vi "geis.vi"(0 "IP adress":string="192.109.209.229", 1 "stop":bool, 2 "Channel":u8(ring) items=["1", "2", "3", "4", "5", "6", "7", "8", "9", "10", "11", "12", "13", "14", "15", "16"], 3 "SGEIS Parameters":T2={"Step_number"=0, "Initial_Current_step"=0.0, "vs_initial "=TRUE, "Final_Current_step"=0.001, "vs_final"=TRUE, "Duration_step"=1.0, "Record_every_dE"=0.1, "Record_every_dT"=0.1, "Initial_frequency"=100000.0, "sweep"=FALSE, "Final_frequency"=1.0, "Frequency_number"=51, "Amplitude_Current"=0.001, "Wait_for_steady"=2.0, "Average_N_times"=1, "Correction"=TRUE, "I_Range"=7, "Bandwidth"=5, "Initial_Current_step 2"=0.01, "vs_initial 2"=FALSE, "em"=1, "ce"=0} {"ce" items=["Standard", "CE to ground"]; "Initial_Current_step" min=-10 max=10 format="%.5f"; "Step_number" min=0 step=1; "Initial_Current_step 2" min=-10 max=10 format="%.5f"; "I_Range" items=["1pA", "1nA", "10nA", "100nA", "1µA", "10µA", "100µA", "1mA", "10mA", "100mA", "1A", "Booster"]; "Bandwidth" items=["1"=1, "2"=2, "3"=3, "4"=4, "5"=5, "6"=6, "7"=7, "8"=8, "9"=9]; "Wait_for_steady" min=0 format="%.2f"; "Record_every_dT" min=0 format="%.2e"; "Record_every_dE" min=0 format="%.2e"; "Duration_step" min=0 format="%.5f"; "Final_Current_step" min=-10 max=10 format="%.5f"; "Average_N_times" min=1 max=1000 step=1; "Amplitude_Current" min=0 max=100 format="%.2e"; "Final_frequency" min=1e-05 max=1000000 format="%.2e"; "Frequency_number" min=1 max=10000; "Initial_frequency" min=1e-05 max=1000000 format="%.2e"}, 4 "Exit":bool, 5 "Start":bool, 8 "Draw":T1(ring)) -> (6 "Number of points":i32=52, 7 "XY Graph":cluster{"Data p1":sgl[], "Data p1":dbl[]}[](graph))   [LabVIEW 2012]
doc: "The Staircase Galvano Electrochemical Impedance Spectroscopy (SGEIS) technique is close to the SPEIS technique, except that the current is controlled instead of the potential.\n\nIn general, in this VI, the first thing to do is to start by establishing the connection with the instrument defined by its IP adress, then load the firmware in the channel selected, get the information on the plugged channels, load protocol on a channel, start/stop the protocol, retreive data and draw the graph.\nThis technique is applied just for channels with impedance capabilities (Zboard)."
uses:
  base_xml.llb/Type Descriptor Enumeration__ogtk.ctl
panel:
  out "Data P0":sgl[][](array[numeric])=[[4.8e-05, 1.2033013, 0.0012545494], [7.2e-05, 4.099232, 0.0030298461], [9.6e-05, 5.4905596, 0.0034574724], [0.00040800002, 5.594096, 0.0031739129], [0.00086400006, 5.697314, 0.00286901], [0.0014160001, 5.800989, 0.0025610582], [0.002112, 5.903515, 0.002253106], [0.0030480002, 6.0050545, 0.0019497279], [0.0045120004, 6.105221, 0.0016379646], [0.008280001, 6.2053866, 0.0013155299], [0.100008, 6.222552, 0.0012118629], [0.200016, 6.223086, 0.0012103383], [0.300024, 6.223086, 0.0012126251], [0.400032, 6.2233143, 0.0012133875], [0.50004, 6.2231617, 0.0012141496], [0.600048, 6.2229333, 0.0012133875], [0.700056, 6.2229333, 0.0012103383], [0.800064, 6.2227044, 0.0012095761], [0.90007204, 6.2233143, 0.0012149118]]
  out "Data P1":sgl[][](array[numeric])=[[99999.99, 0.015896028, 2.4134535e-05, -0.31541085, 6.2027836, 0.0012093844, 0.0, 0.028001478, 2.4202996e-05, -0.21167731, -6.8013325, -0.001209385, 0.0, 1.296, 8.0], [79789.055, 0.020694803, 3.145496e-05, -0.31517792, 6.1967587, 0.0012085777, 0.0, 0.036134787, 3.1510877e-05, -0.20527963, -6.7949142, -0.0012085784, 0.0, 1.584, 8.0], [63671.867, 0.027115118, 3.95239e-05, -0.36039186, 6.1889963, 0.0012069115, 0.0, 0.04638151, 3.95688e-05, -0.23149349, -6.7864842, -0.0012069122, 0.0, 1.872, 8.0], [50804.684, 0.035882276, 4.949095e-05, -0.40444195, 6.178996, 0.0012048192, 0.0, 0.05973892, 4.952679e-05, -0.25926352, -6.77554, -0.0012048199, 0.0, 2.16, 8.0], [40539.06, 0.048188828, 6.136454e-05, -0.4440093, 6.1657524, 0.0012020994, 0.0, 0.077702746, 6.139315e-05, -0.28762102, -6.7610307, -0.0012021001, 0.0, 2.448, 8.0], [32343.752, 0.06770085, 7.88223e-05, -0.47251844, 6.1465006, 0.0011982684, 0.0, 0.10554845, 7.884587e-05, -0.31181583, -6.739913, -0.0011982691, 0.0, 2.736, 8.0], [25812.496, 0.12644306, 0.0001329111, -0.48514298, 6.0997047, 0.0011887155, 0.0, 0.19051811, 0.00013293685, -0.32698154, -6.6886125, -0.0011887162, 0.0, 3.024, 8.0], [20593.748, 0.23297587, 0.00022114319, -0.47706103, 6.015843, 0.0011718888, 0.0, 0.34030145, 0.00022117054, -0.3275948, -6.596549, -0.0011718895, 0.0, 3.312, 8.0], [16429.69, 0.37617812, 0.00032387703, -0.45101714, 5.8985395, 0.0011485365, 0.0, 0.5348972, 0.00032390282, -0.31515712, -6.4677424, -0.0011485372, 0.0, 3.6000001, 8.0], [13109.373, 0.55603534, 0.00044012873, -0.4103434, 5.7451816, 0.0011180385, 0.0, 0.7737537, 0.00044015126, -0.2906543, -6.299325, -0.0011180392, 0.0, 3.888, 8.0], [10460.936, 0.7749276, 0.00057313335, -0.36184657, 5.5526934, 0.001079828, 0.0, 1.0605142, 0.0005731519, -0.25886726, -6.0878835, -0.0010798287, 1.0, 4.176, 8.0], [8351.5625, 1.0352163, 0.00072714745, -0.31150156, 5.3164287, 0.0010371187, 1.0, 1.3994575, 0.0007271621, -0.22451091, -5.8299828, -0.0010371194, 1.0, 4.609, 8.0], [6660.1553, 1.3410046, 0.000907536, -0.26282227, 5.0436444, 0.0009789959, 1.0, 1.7970788, 0.00090754736, -0.19028175, -5.5293727, -0.0009789965, 2.0, 4.947, 8.0], [5313.953, 1.5113798, 0.0009967732, -0.21961367, 4.8940244, 0.0009556693, 1.0, 2.0129824, 0.000996781, -0.15885389, -5.3671427, -0.00095566985, 2.0, 5.57, 8.0], [4241.786, 1.5454612, 0.0010015898, -0.18297291, 4.878454, 0.0009537674, 1.0, 2.0500069, 0.0010015944, -0.13264023, -5.3505425, -0.0009537679, 2.0, 6.213, 8.0], [3385.4163, 1.5790181, 0.0010115571, -0.153041, 4.8648095, 0.00095176516, 1.0, 2.0889149, 0.0010115607, -0.111195564, -5.3358197, -0.0009517657, 2.0, 6.857, 8.0], [2699.3184, 1.5802759, 0.0010046018, -0.1293776, 4.883166, 0.0009544167, 1.0, 2.0867875, 0.0010046042, -0.09421384, -5.3556128, -0.0009544172, 2.0, 7.501, 8.0], [2153.4448, 1.5856456, 0.001002952, -0.11168504, 4.8972144, 0.0009564839, 1.0, 2.0912726, 0.0010029528, -0.08150327, -5.370766, -0.0009564844, 2.0, 8.1449995, 8.0], [1717.748, 1.5895984, 0.0010019304, -0.09921706, 4.9112163, 0.0009589054, 1.0, 2.0948448, 0.0010019315, -0.072561264, -5.38597, -0.0009589059, 2.0, 8.792, 8.0], [1372.1951, 1.5920151, 0.0010009218, -0.09178877, 4.924607, 0.0009613617, 1.0, 2.0966747, 0.0010009219, -0.06731814, -5.400561, -0.0009613622, 2.0, 9.439, 8.0], [1096.7545, 1.6009942, 0.0010047532, -0.08871567, 4.9333324, 0.000961253, 1.0, 2.1073825, 0.001004754, -0.06525302, -5.4094787, -0.00096125354, 2.0, 9.871, 8.0], [871.93097, 1.5816059, 0.0009906995, -0.09027839, 4.959241, 0.000966918, 1.0, 2.0806665, 0.0009906992, -0.06663093, -5.4381466, -0.00096691854, 2.0, 10.307, 8.0], [696.1138, 1.5729876, 0.0009832102, -0.09623489, 4.9737277, 0.0009698118, 1.0, 2.0679011, 0.0009832109, -0.07122159, -5.454079, -0.0009698124, 2.0, 10.741, 8.0], [555.8894, 1.6019666, 0.0009985057, -0.106960624, 4.9539285, 0.00096688373, 1.0, 2.1039863, 0.0009985064, -0.07941079, -5.4326506, -0.0009668843, 2.0, 11.394, 8.0], [443.43906, 1.6082691, 0.0009985616, -0.122988224, 4.9526095, 0.0009666943, 1.0, 2.1093283, 0.000998562, -0.091551304, -5.4311996, -0.00096669485, 2.0, 12.053, 8.0], [353.75473, 1.6163155, 0.0009975499, -0.14474046, 4.9489985, 0.00096599624, 1.0, 2.1154938, 0.0009975497, -0.10804355, -5.427236, -0.0009659968, 2.0, 12.715, 8.0], [281.8943, 1.6319947, 0.000997945, -0.1731171, 4.939253, 0.000964064, 1.0, 2.1291127, 0.0009979454, -0.12966967, -5.416549, -0.00096406456, 2.0, 13.377, 8.0], [225.3606, 1.6545873, 0.000997958, -0.20826769, 4.9249706, 0.00096138736, 1.0, 2.1484613, 0.0009979575, -0.15665877, -5.4009104, -0.0009613879, 2.0, 14.045, 8.0], [180.28844, 1.6867937, 0.0009969639, -0.25068158, 4.9050946, 0.0009575135, 1.0, 2.1753373, 0.0009969644, -0.18979812, -5.3791265, -0.0009575141, 2.0, 14.722, 8.0], [143.75787, 1.7397344, 0.0009973684, -0.30079174, 4.872224, 0.00095120573, 1.0, 2.2215395, 0.0009973678, -0.22964483, -5.3430943, -0.0009512063, 2.0, 15.411, 8.0], [114.59661, 1.8171204, 0.0009974693, -0.3567279, 4.8248806, 0.00094198145, 1.0, 2.2893379, 0.0009974696, -0.27555776, -5.2911463, -0.00094198197, 2.0, 16.109, 8.0], [91.552734, 1.9272654, 0.0009971086, -0.4146781, 4.7582307, 0.00092904264, 2.0, 2.3872557, 0.0009971082, -0.32522857, -5.217652, -0.00092904316, 2.0, 17.039999, 8.0], [72.87778, 2.0835702, 0.0009966118, -0.47080094, 4.6631265, 0.00091063714, 2.0, 2.5288415, 0.0009966121, -0.37639964, -5.1133604, -0.00091063767, 2.0, 17.782999, 8.0], [58.30223, 2.290216, 0.0009965424, -0.5163753, 4.536835, 0.00088618894, 2.0, 2.7210877, 0.000996542, -0.42156878, -4.9748783, -0.00088618946, 2.0, 18.546999, 8.0], [46.50297, 2.5567615, 0.0009965401, -0.54690737, 4.373813, 0.0008546952, 2.0, 2.9750876, 0.0009965405, -0.45663965, -4.796084, -0.00085469574, 2.0, 19.302, 8.0], [36.95101, 2.8818939, 0.0009962525, -0.55650496, 4.17603, 0.0008164121, 2.0, 3.292113, 0.0009962524, -0.47500235, -4.5792, -0.00081641256, 2.0, 20.077, 8.0], [29.592804, 3.234223, 0.0009962742, -0.5438912, 3.963954, 0.0007754039, 2.0, 3.6432135, 0.000996275, -0.47317147, -4.346668, -0.0007754044, 2.0, 20.93, 8.0], [23.588463, 3.6068342, 0.0009961284, -0.5106709, 3.7440598, 0.0007329593, 2.0, 4.0214486, 0.0009961289, -0.45162058, -4.1054997, -0.0007329597, 2.0, 21.862, 8.0], [18.780045, 3.9640598, 0.0009960186, -0.46161065, 3.5391219, 0.00069332117, 2.0, 4.3898535, 0.0009960192, -0.41360545, -3.8807545, -0.0006933216, 2.0, 22.863, 8.0], [15.024037, 4.271375, 0.0009959555, -0.40523124, 3.3689148, 0.00066039263, 2.0, 4.710784, 0.0009959557, -0.36663783, -3.694098, -0.00066039304, 2.0, 23.906, 8.0], [11.982363, 4.520932, 0.0009950611, -0.3458606, 3.2371411, 0.0006348915, 2.0, 4.9737754, 0.000995061, -0.31517577, -3.5495536, -0.0006348918, 2.0, 24.949, 8.0], [9.574144, 2.38077, 0.0005031747, -0.28917873, 4.6680098, 0.0009119648, 2.0, 2.6153588, 0.0005031747, -0.26482016, -5.1187296, -0.00091196527, 2.0, 25.382, 8.0], [7.6293964, 2.4353614, 0.0004999304, -0.23806715, 4.644746, 0.0009074361, 2.0, 2.6731777, 0.00049993006, -0.21878657, -5.0931625, -0.0009074366, 2.0, 25.922, 8.0], [6.084501, 2.4750657, 0.00049832056, -0.19374752, 4.6285977, 0.0009043441, 2.0, 2.7155764, 0.0004983205, -0.17844573, -5.075479, -0.0009043446, 2.0, 26.594, 8.0], [4.858519, 2.5030587, 0.0004974475, -0.15684187, 4.617654, 0.0009022134, 2.0, 2.7455964, 0.0004974477, -0.14467418, -5.0634913, -0.000902214, 2.0, 27.432001, 8.0], [3.8752477, 2.52257, 0.0004969658, -0.12630916, 4.6102643, 0.0009008552, 2.0, 2.7666035, 0.00049696607, -0.11720729, -5.055331, -0.00090085575, 2.0, 28.479, 8.0], [3.1001983, 2.5355425, 0.0004967685, -0.101694584, 4.6055255, 0.0008999815, 2.0, 2.7805579, 0.0004967687, -0.09457946, -5.050148, -0.000899982, 2.0, 29.784, 8.0], [2.4660668, 2.5443485, 0.00049676636, -0.0811795, 4.602378, 0.0008993778, 2.0, 2.7900364, 0.00049676653, -0.075683355, -5.046685, -0.0008993783, 2.0, 31.421001, 8.0], [1.9649143, 2.550054, 0.0004967066, -0.06482482, 4.600377, 0.0008989733, 2.0, 2.7961702, 0.0004967067, -0.060593843, -5.0444574, -0.00089897384, 2.0, 33.471, 8.0], [1.5725644, 2.5537558, 0.0004967495, -0.051944494, 4.599086, 0.00089873036, 2.0, 2.8001752, 0.0004967496, -0.04870844, -5.043045, -0.0008987309, 2.0, 36.029, 8.0], [1.2520034, 2.5562146, 0.00049671344, -0.04138118, 4.5982056, 0.00089857634, 2.0, 2.8028417, 0.00049671356, -0.03896928, -5.042108, -0.00089857687, 2.0, 39.239, 8.0], [1.0016024, 2.557709, 0.00049671053, -0.03315392, 4.597694, 0.0008984848, 2.0, 2.8044465, 0.00049671077, -0.031377077, -5.0415564, -0.00089848536, 2.0, 43.248, 8.0]]
  out "Exit 2":bool=TRUE
  # "Instructions:\nBefore running the VI you must type a valid IP adress that corresponds to the instrument.Then press the Run button to execute this VI.\nWhile this VI is running, choose the available channel, enter the SGEIS parameters or keep the default\n values, then press the button start to begin the experience. \nChoose the waveform to draw : Nyquist, modZ, theta...\nPress the stop button to end experience and the exit button to stop the VI execution."
  # "Set I (A)  vs. previous"
  # "Set I (A)  vs. previous"
  # "Before EIS  stay for ts (s)"
  # "and record every dE (V)"
  # "or every dt (s)"
  # "Start EIS from  Fi (Hz)"
  # "sweep linear/logarithmic"
  # "to Ff (Hz)"
  # "for Nf frequencies"
  # "with the amplitude (A)"
  # "wait for Pw"
  # "average Na times"
  # "drift correction"
  # "with I Range"
  # "bandwidth"
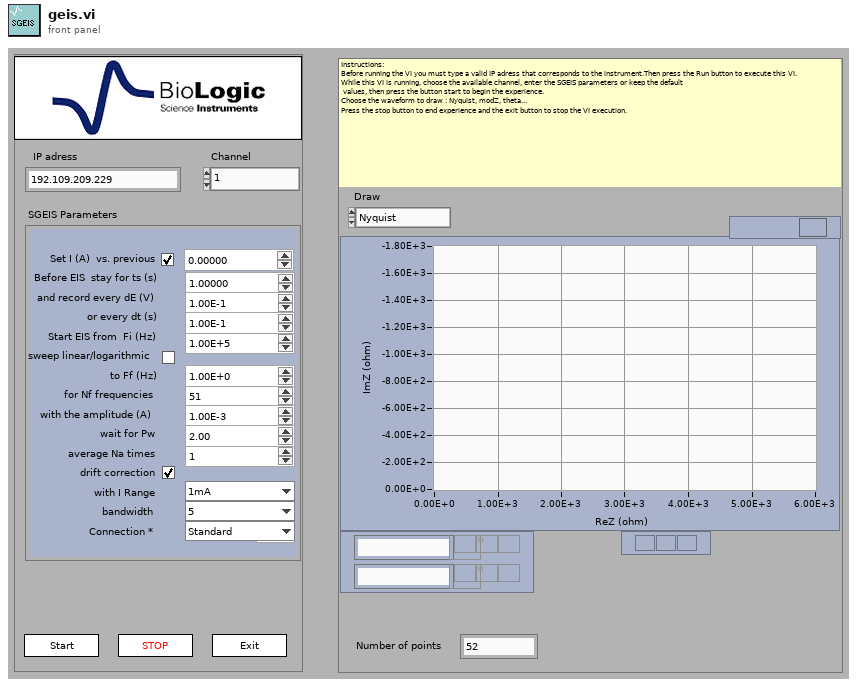
[diagram p1: front panel]
types:
  T1 = enum16{"Nyquist", "modZ", "theta", "modE", "modI", "Edc", "Idc", "E range", "I range", "f(t)"}
  T2 = cluster{"Step_number":i32, "Initial_Current_step":sgl, "vs_initial ":bool, "Final_Current_step":sgl, "vs_final":bool, "Duration_step":sgl, "Record_every_dE":sgl, "Record_every_dT":sgl, "Initial_frequency":sgl, "sweep":bool, "Final_frequency":sgl, "Frequency_number":i32, "Amplitude_Current":sgl, "Wait_for_steady":sgl, "Average_N_times":i32, "Correction":bool, "I_Range":u16, "Bandwidth":u16, "Initial_Current_step 2":sgl, "vs_initial 2":bool, "em":u16, "ce":u16}
  T3 = typedef "Type Descriptor Enumeration__ogtk.ctl" = enum8{"<Null>", "I8", "I16", "I32", "I64", "U8", "U16", "U32", "U64", "SGL", "DBL", "EXT", "CSG", "CDB", "CXT", "0x0F", "0x10", "0x11", "0x12", "0x13", "0x14", "Enum U8", "Enum U16", "Enum U32", "Enum U64", "SGL PQ", "DBL PQ", "EXT PQ", "CSG PQ", "CDB PQ", "CXT PQ", "0x1F", "0x20", "Boolean", "0x22", "0x23", "0x24", "0x25", "0x26", "0x27", "0x28", "0x29", "0x2A", "0x2B", "0x2C", "0x2D", "0x2E", "0x2F", "String", "0x31", "Path", "Pict", "0x34", "0x35", "0x36", "DAQ", "0x38", "0x39", "0x3A", "0x3B", "0x3C", "0x3D", "0x3E", "0x3F", "Array", "0x41", "0x42", "0x43", "0x44", "0x45", "0x46", "0x47", "0x48", "0x49", "0x4A", "0x4B", "0x4C", "0x4D", "0x4E", "0x4F", "Cluster", "0x51", "0x52", "Variant", "Waveform", "0x55", "0x56", "0x57", "0x58", "0x59", "0x5A", "0x5B", "0x5C", "0x5D", "0x5E", "0x5F", "0x60", "0x61", "0x62", "0x63", "0x64", "0x65", "0x66", "0x67", "0x68", "0x69", "0x6A", "0x6B", "0x6C", "0x6D", "0x6E", "0x6F", "Refnum"}
  T4 = cluster{"Data Type":T3, "Format String":string}[]
  T5 = cluster{"Channel":i32, "BoardVersion":i32, "BoardSerialCode":i32, "FirmwareCode":i32, "FirmwareVersion":i32, "XilinxVersion":i32, "AmpCode":i32, "NbAmp":i32, "LcBoard":i32, "Zboard":i32, "MuxBoard":i32, "GPRAboard":i32, "MemSize":i32, "MemFilled":i32, "state":i32, "MaxIRange":i32, "MinIRange":i32, "MaxBandwidth":i32, "NbOfTechniques":i32}
  T6 = cluster{"Label":string, "type":i32, "valeur":u32, "index":i32}[]
  T7 = cluster{"IRQskipped":i32, "NbRaws":i32, "NbCols":i32, "Technique Index":i32, "TechniqueID":i32, "PrcessIndex":i32, "loop":i32, "StartTime":dbl, "MuxPad":i32}
  T8 = cluster{"State":i32, "MemFilled":i32, "TimeBase":sgl, " Ewe":sgl, " EweRangeMin":sgl, " EweRangeMax":sgl, "Ece":sgl, "EceRangeMin":sgl, "EceRangeMax":sgl, "Eoverflow":i32, "I":sgl, "IRange":i32, "Ioverflow":i32, "ElapsedTime":sgl, "Freq":sgl, "Rcomp":sgl, "Saturation":sgl, "OptErr":i32, "OptPos":i32}
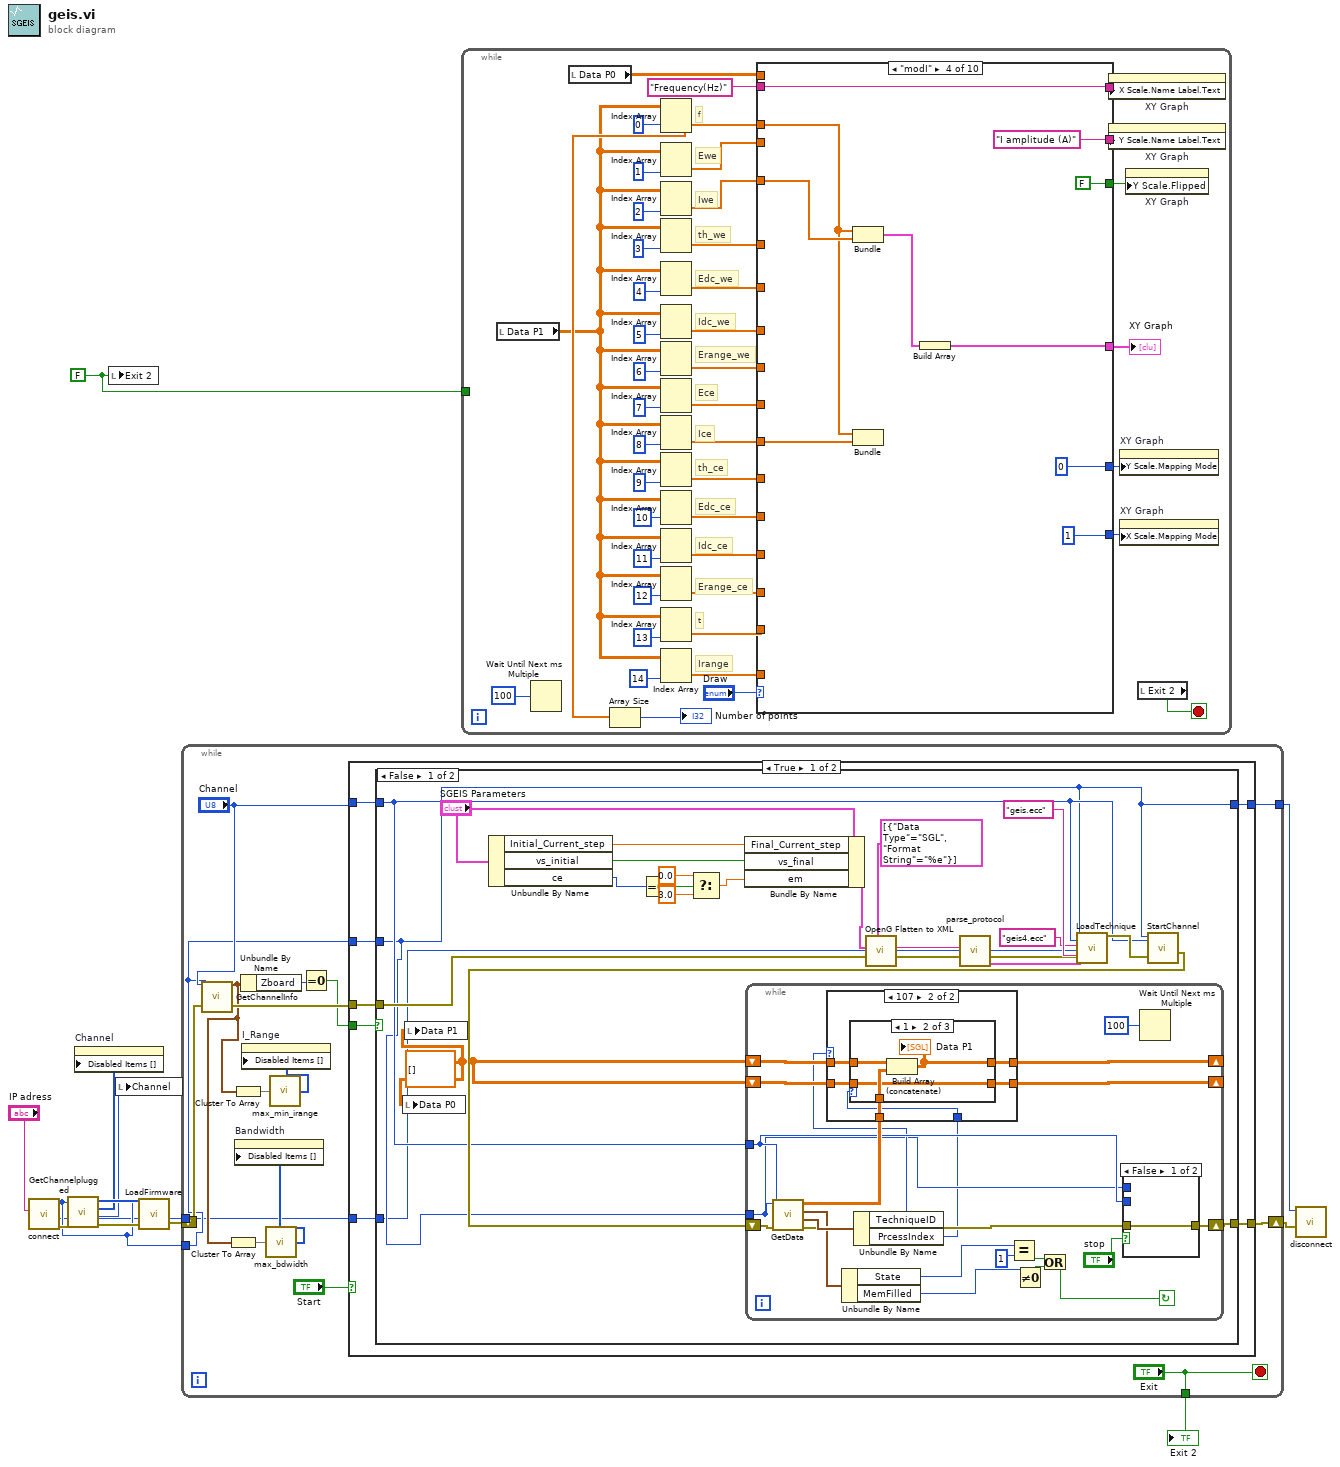
[diagram p0: block diagram]
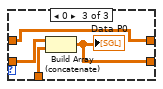
[diagram p4: hidden frame]
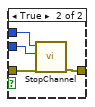
[diagram p5: hidden frame]
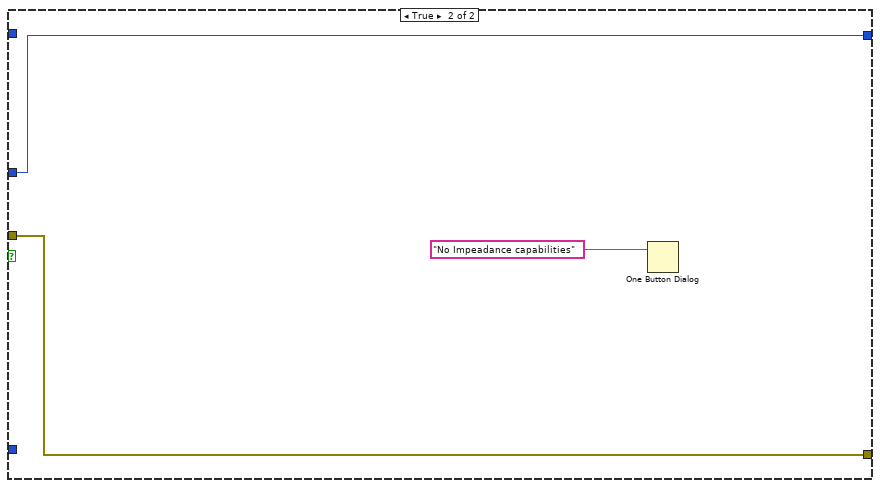
[diagram p6: hidden frame]
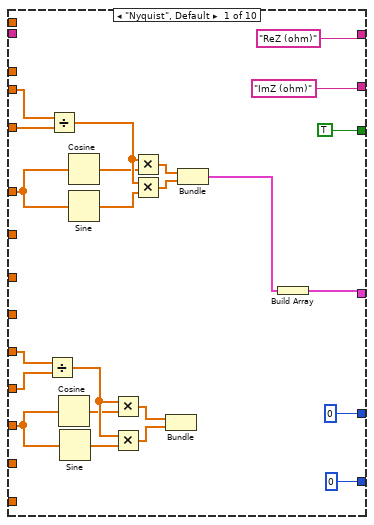
[diagram p8: hidden frame]
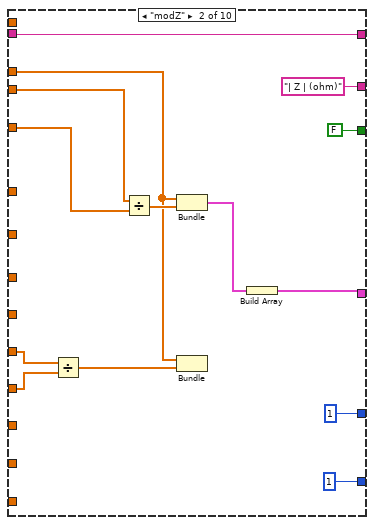
[diagram p9: hidden frame]
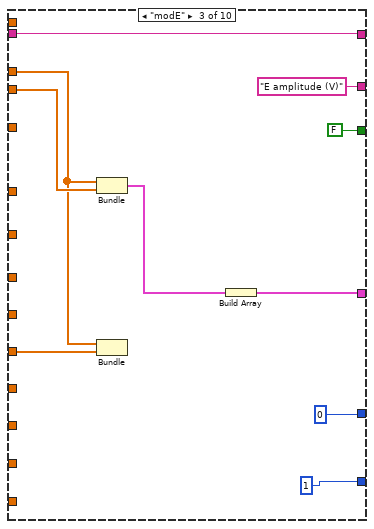
[diagram p10: hidden frame]
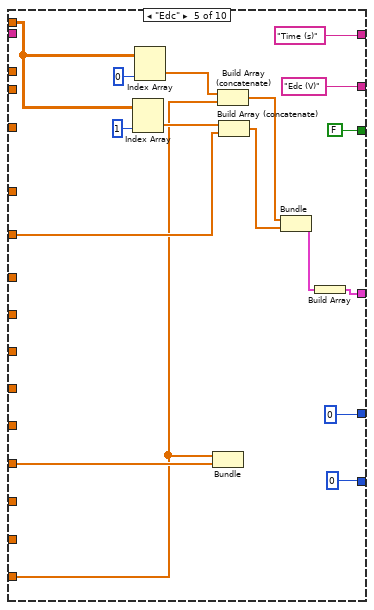
[diagram p11: hidden frame]
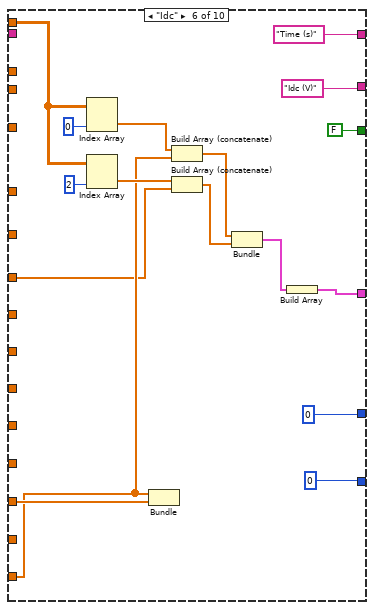
[diagram p12: hidden frame]
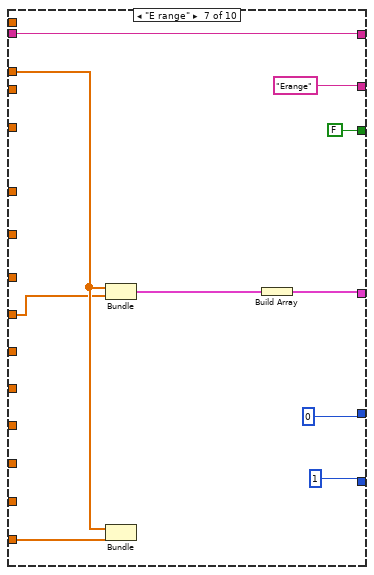
[diagram p13: hidden frame]
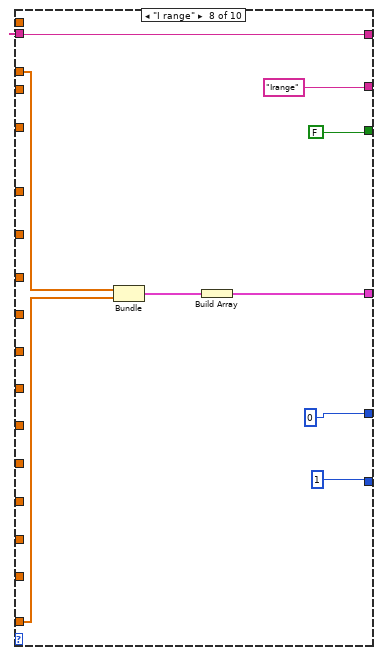
[diagram p14: hidden frame]
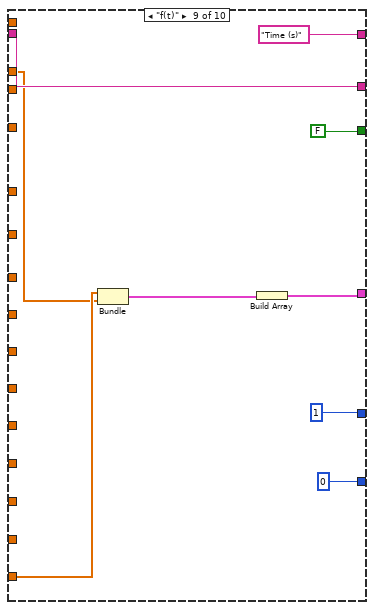
[diagram p15: hidden frame]
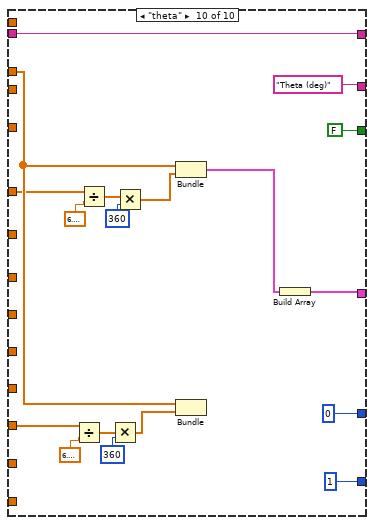
[diagram p16: hidden frame]
diagram:
  w6 = FALSE
  n1 = call "connect.vi"("IP"="IP adress") -> ("error out"=w12:errorcluster, "Device Code"=w1:i32, "ID"=w3:i32)  [unwired: 7 in, 1 out]
  n2 = call "GetChannelplugged.vi"("error in (no error)"=w12, "ID"=w3) -> ("error out"=w10:errorcluster, "First channel"=w8:i32, "Disabled channels"=w7:i32[], "Plugged channels"=w11:i32[])  [unwired: 6 in]
  n3 = property on="Channel" class="Ring (strict)"("Disabled Items []"=w7) -> ()  [unwired: 2 in, 2 out]
  n4 = local write "Exit 2"(w6) -> ()
  n5 = local write "Channel"(w8) -> ()
  n6 = call "LoadFirmware.vi"("error in (no error)"=w10, "Channels"=w11, "ID"=w3) -> ("error out"=w4:errorcluster)  [unwired: 7 in, 1 out]
  n7 = while {
    shift-right: [w28] -> w13
    shift-left: w4 -> [w23]
    tunnel: ["Exit"] -> w5
    tunnel: w3 -> [w18]
    tunnel: [w17] -> w2
    tunnel: w1 -> [w14]
    stop <- "Exit" stop-if-true
    n8 = call "GetChannelInfo.vi"("error in (no error)"=w23, "Channel"="Channel", "ID"=w18) -> ("error out"=w24:errorcluster, "Channel information"=w19:T5)  [unwired: 7 in]
    n9 = Cluster To Array(cluster=w19) -> (array=w20:i32[])
    n10 = Cluster To Array(cluster=w19) -> (array=w21:i32[])
    n11 = Unbundle By Name(w19) -> ("Zboard"=w26:i32)
    n12 = call "max_bdwidth.vi"("resources"=w20) -> ("disabled ranges"=w16:i32[])
    n13 = property on="Bandwidth" class="Ring (strict)"("Disabled Items []"=w16) -> ()  [unwired: 2 in, 2 out]
    n14 = call "max_min_irange.vi"("resources"=w21) -> ("disabled ranges"=w15:i32[])
    n15 = property on="I_Range" class="Ring (strict)"("Disabled Items []"=w15) -> ()  [unwired: 2 in, 2 out]
    n16 = Equal To 0?(x=w26) -> (x = 0?=w22:bool)
    n17 = case shown="True" "Start" {
      tunnel: "Channel" -> [w35 _]
      tunnel: [w36 w108] -> w28
      tunnel: w24 -> [w34 w108]
      tunnel: w22 -> [w33 _]
      tunnel: w18 -> [w32 w107]
      tunnel: [w31 w107] -> w17
      tunnel: w14 -> [w30 _]
      frame True {
        n18 = case shown="False" w33 {
          tunnel: [w55 w105] -> w36
          tunnel: w35 -> [w53 _]
          tunnel: w34 -> [w54 w105]
          tunnel: w32 -> [w49 w104]
          tunnel: [w49 w104] -> w31
          tunnel: w30 -> [w47 _]
          frame False {
            w52 = sgl[][] [] ("Data")
            n19 = local write "Data P0"(w52) -> ()
            n20 = local write "Data P1"(w52) -> ()
            n21 = Unbundle By Name("SGEIS Parameters") -> ("Initial_Current_step"=w45:sgl, "vs_initial"=w44:bool, "ce"=w38:u16)
            n22 = Equal To 0?(x=w38) -> (x = 0?=w39:bool)
            n23 = Select(t=0.0, s=w39, f=3.0) -> (s? t:f=w37:dbl)
            n24 = Bundle By Name(cluster="SGEIS Parameters", "Final_Current_step"=w45, "vs_final"=w44, "em"=w37) -> (w42:T2)
            n25 = call "OpenG Flatten to XML.vi"("Type Formats (default)"=T4 [{"Data Type"=enum."SGL", "Format String"="%e"}] ("Type Formats"), "LabVIEW Data"=w42) -> ("XML String"=w50:string)  [unwired: 8 in, 1 out]
            n26 = call "parse_protocol.vi"("XML String In"=w50) -> ("Params Values"=w48:T6)  [unwired: 8 in]
            n27 = call "LoadTechnique.vi"("ID"=w49, "Selected Channel"=w53, "FName4"="geis4.ecc" ("FName"), "Device Code"=w47, "FName"="geis.ecc", "Protocol Parameters"=w48, "error in (no error)"=w54) -> ("error out"=w57:errorcluster)  [unwired: 12 in]
            n28 = call "StartChannel.vi"("error in (no error)"=w57, "Channel"=w53, "ID"=w49) -> ("error out"=w56:errorcluster)  [unwired: 8 in]
            n29 = while {
              shift-right: [w74] -> w55
              shift-left: w56 -> [w76]
              tunnel: w53 -> [w65]
              shift-right: [w70] -> _
              shift-left: w52 -> [w71]
              shift-right: [w68] -> _
              shift-left: w52 -> [w69]
              tunnel: w49 -> [w63]
              stop <- w72 continue-if-true
              n30 = call "GetData.vi"("error in (no error)"=w76, "Channel"=w65, "ID"=w63) -> ("error out"=w73:errorcluster, "Data information"=w80:T7, "Current values"=w62:T8, "Data"=w67:dbl[][])  [unwired: 5 in]
              n31 = Unbundle By Name(w62) -> ("State"=w61:i32, "MemFilled"=w60:i32)
              n32 = Unbundle By Name(w80) -> ("TechniqueID"=w64:i32, "PrcessIndex"=w59:i32)
              n33 = case shown="107" w64 {
                tunnel: w71 -> [w82 w88]
                tunnel: [w82 w87] -> w70
                tunnel: w69 -> [w81 w86]
                tunnel: [w81 w85] -> w68
                tunnel: w67 -> [_ w84]
                tunnel: w59 -> [_ w83]
                frame 0, Default {
                }
                frame 107 {
                  n34 = case shown="1" w83 {
                    tunnel: [w90 w92 w95] -> w87
                    tunnel: w88 -> [w90 w93 w95]
                    tunnel: [w89 w91 w96] -> w85
                    tunnel: w86 -> [w89 w91 w98]
                    tunnel: w84 -> [_ w94 w97]
                    frame 2, Default {
                    }
                    frame 1 {
                      n35 = Build Array (concatenate)(w93, w94) -> (w92:dbl[][])
                      "Data P1" <- w92
                    }
                    frame 0 {
                      n36 = Build Array (concatenate)(w98, w97) -> (w96:dbl[][])
                      "Data P0" <- w96
                    }
                  }
                }
              }
              n37 = Equal?(x=w61, y=1) -> (x = y?=w78:bool)
              n38 = Not Equal To 0?(x=w60) -> (x != 0?=w77:bool)
              n39 = Or(x=w78, y=w77) -> (x .or. y?=w72:bool)
              n40 = case shown="False" "stop" {
                tunnel: [w99 w103] -> w74
                tunnel: w73 -> [w99 w102]
                tunnel: w65 -> [_ w101]
                tunnel: w63 -> [_ w100]
                frame False {
                }
                frame True {
                  n41 = call "StopChannel.vi"("error in (no error)"=w102, "Channel"=w101, "ID"=w100) -> ("error out"=w103:errorcluster)  [unwired: 8 in]
                }
              }
              n42 = Wait Until Next ms Multiple(millisecond multiple=u32 100) -> ()  [unwired: 1 out]
            }
          }
          frame True {
            n43 = One Button Dialog(message="No Impeadance capabilities" ("error source (\" \")")) -> ()  [unwired: 1 in, 1 out]
          }
        }
      }
      frame False {
      }
    }
  }
  "Exit 2" <- w5
  n44 = while {
    tunnel: w6 -> [_]
    stop <- w140 stop-if-true
    # "Erange_ce"
    # "Idc_ce"
    # "Edc_ce"
    # "th_ce"
    # "Ice"
    # "Ece"
    # "t"
    # "Irange"
    # "Erange_we"
    # "Idc_we"
    # "Edc_we"
    # "th_we"
    # "Iwe"
    # "Ewe"
    # "f"
    n45 = local read "Data P1"() -> (w110:sgl[][])
    n46 = Wait Until Next ms Multiple(millisecond multiple=u32 100) -> ()  [unwired: 1 out]
    n47 = local read "Data P0"() -> (w109:sgl[][])
    n48 = Index Array(array=w110, index (col)=0 ("Index")) -> (element=w124:sgl[])  [unwired: 1 in]
    n49 = Array Size(array=w124) -> (size(s)=→"Number of points":i32)
    n50 = Index Array(array=w110, index (col)=1 ("Index")) -> (element=w125:sgl[])  [unwired: 1 in]
    n51 = Index Array(array=w110, index (col)=2 ("Index")) -> (element=w130:sgl[])  [unwired: 1 in]
    n52 = Index Array(array=w110, index (col)=3 ("Index")) -> (element=w145:sgl[])  [unwired: 1 in]
    n53 = Index Array(array=w110, index (col)=4 ("disabled index (col)")) -> (element=w139:sgl[])  [unwired: 1 in]
    n54 = Index Array(array=w110, index (col)=5 ("disabled index (col)")) -> (element=w136:sgl[])  [unwired: 1 in]
    n55 = Index Array(array=w110, index (col)=6 ("index (row)")) -> (element=w126:sgl[])  [unwired: 1 in]
    n56 = Index Array(array=w110, index (col)=7) -> (element=w117:sgl[])  [unwired: 1 in]
    n57 = Index Array(array=w110, index (col)=8) -> (element=w116:sgl[])  [unwired: 1 in]
    n58 = Index Array(array=w110, index (col)=9) -> (element=w115:sgl[])  [unwired: 1 in]
    n59 = Index Array(array=w110, index (col)=10) -> (element=w114:sgl[])  [unwired: 1 in]
    n60 = Index Array(array=w110, index (col)=11) -> (element=w113:sgl[])  [unwired: 1 in]
    n61 = Index Array(array=w110, index (col)=12) -> (element=w112:sgl[])  [unwired: 1 in]
    n62 = Index Array(array=w110, index (col)=13 ("disabled index (col)")) -> (element=w127:sgl[])  [unwired: 1 in]
    n63 = Index Array(array=w110, index (col)=14 ("disabled index (col)")) -> (element=w128:sgl[])  [unwired: 1 in]
    n64 = case shown="\"modI\"" "Draw" {
      tunnel: w124 -> [_ w181 w191 w202 _ _ w247 w255 w264 w275]
      tunnel: w125 -> [w157 w179 w198 _ _ _ _ _ _ _]
      tunnel: w130 -> [w156 w178 _ w208 _ _ _ _ _ _]
      tunnel: ["ImZ (ohm)" ("Y Scale.Name Label.Text") "| Z | (ohm)" ("Y Scale.Name Label.Text") "E amplitude (V)" ("Y Scale.Name Label.Text") "I amplitude (A)" ("Y Scale.Name Label.Text") "Edc (V)" ("Y Scale.Name Label.Text") "Idc (V)" ("Y Scale.Name Label.Text") "Erange" ("Y Scale.Name Label.Text") "Irange" ("Y Scale.Name Label.Text") w269 "Theta (deg)" ("Y Scale.Name Label.Text")] -> w147
      tunnel: w145 -> [w152 _ _ _ _ _ _ _ _ w273]
      tunnel: ["ReZ (ohm)" ("Y Scale.Name Label.Text") w186 w196 w206 "Time (s)" ("Y Scale.Name Label.Text") "Time (s)" ("Y Scale.Name Label.Text") w252 w261 "Time (s)" ("Y Scale.Name Label.Text") w288] -> w144
      tunnel: "Frequency(Hz)" ("Y Scale.Name Label.Text") -> [_ w186 w196 w206 _ _ w252 w261 w269 w288]
      tunnel: [TRUE ("Y Scale.Flipped") FALSE ("Y Scale.Flipped") FALSE ("Y Scale.Flipped") FALSE ("Y Scale.Flipped") FALSE ("Y Scale.Flipped") FALSE ("Y Scale.Flipped") FALSE ("Y Scale.Flipped") FALSE FALSE FALSE ("Y Scale.Flipped")] -> w142
      tunnel: [u8 0 ("X Scale.Mapping Mode") u8 1 ("X Scale.Mapping Mode") u8 1 ("X Scale.Mapping Mode") u8 1 ("X Scale.Mapping Mode") 0 0 1 1 0 u8 1 ("X Scale.Mapping Mode")] -> w141
      tunnel: w139 -> [_ _ _ _ w213 _ _ _ _ _]
      tunnel: w136 -> [_ _ _ _ _ w227 _ _ _ _]
      tunnel: w126 -> [_ _ _ _ _ _ w244 _ _ _]
      tunnel: w128 -> [_ _ _ _ _ _ _ w256 _ _]
      tunnel: w127 -> [_ _ _ _ w210 w228 _ _ w265 _]
      tunnel: [0 1 u8 0 ("X Scale.Mapping Mode") u8 0 ("X Scale.Mapping Mode") 0 0 0 0 1 0 ("X Scale.Mapping Mode")] -> w132
      tunnel: w117 -> [w155 w177 w192 _ _ _ _ _ _ _]
      tunnel: w116 -> [w154 w176 _ w201 _ _ _ _ _ _]
      tunnel: w115 -> [w153 _ _ _ _ _ _ _ _ w272]
      tunnel: w114 -> [_ _ _ _ w212 _ _ _ _ _]
      tunnel: w113 -> [_ _ _ _ _ w229 _ _ _ _]
      tunnel: w112 -> [_ _ _ _ _ _ w245 _ _ _]
      tunnel: [w162 w175 w189 w199 w211 w230 w243 w253 w262 w271] -> w111
      tunnel: w109 -> [_ _ _ _ w214 w231 _ _ _ _]
      frame "Nyquist", Default {
        n65 = Divide(x=w155, y=w154) -> (x/y=w159:sgl[])
        n66 = Divide(x=w157, y=w156) -> (x/y=w161:sgl[])
        n67 = Cosine(x=w153) -> (cos(x)=w158:sgl[])
        n68 = Sine(x=w153) -> (sin(x)=w164:sgl[])
        n69 = Cosine(x=w152) -> (cos(x)=w160:sgl[])
        n70 = Sine(x=w152) -> (sin(x)=w174:sgl[])
        n71 = Multiply(x=w159, y=w158) -> (x*y=w166:sgl[])
        n72 = Multiply(x=w159, y=w164) -> (x*y=w165:sgl[])
        n73 = Multiply(x=w161, y=w160) -> (x*y=w168:sgl[])
        n74 = Multiply(x=w161, y=w174) -> (x*y=w169:sgl[])
        n75 = Bundle(w166, w165) -> ()  [unwired: 1 in, 1 out]
        n76 = Bundle(w168, w169) -> (w163:cluster{sgl[], sgl[]})  [unwired: 1 in]
        n77 = Build Array(w163) -> (w162:cluster{sgl[], sgl[]}[])
      }
      frame "modZ" {
        n78 = Divide(x=w177, y=w176) -> (x/y=w182:sgl[])
        n79 = Divide(x=w179, y=w178) -> (x/y=w188:sgl[])
        n80 = Bundle("Data P1"=w181, w188) -> (w180:cluster{"Data P1":sgl[], sgl[]})  [unwired: 1 in]
        n81 = Bundle("Data P1"=w181, w182) -> ()  [unwired: 1 in, 1 out]
        n82 = Build Array(w180) -> (w175:cluster{"Data P1":sgl[], sgl[]}[])
      }
      frame "modE" {
        n83 = Bundle("Data P1"=w191, "Data P1"=w198) -> (w190:cluster{"Data P1":sgl[], "Data P1":sgl[]})  [unwired: 1 in]
        n84 = Bundle("Data P1"=w191, "Data P1"=w192) -> ()  [unwired: 1 in, 1 out]
        n85 = Build Array(w190) -> (w189:cluster{"Data P1":sgl[], "Data P1":sgl[]}[])
      }
      frame "modI" {
        n86 = Bundle("Data P1"=w202, "Data P1"=w208) -> (w200:cluster{"Data P1":sgl[], "Data P1":sgl[]})  [unwired: 1 in]
        n87 = Bundle("Data P1"=w202, "Data P1"=w201) -> ()  [unwired: 1 in, 1 out]
        n88 = Build Array(w200) -> (w199:cluster{"Data P1":sgl[], "Data P1":sgl[]}[])
      }
      frame "Edc" {
        n89 = Index Array(array=w214, index (col)=1 ("Index")) -> (element=w215:sgl[])  [unwired: 1 in]
        n90 = Index Array(array=w214, index (col)=0 ("Index")) -> (element=w216:sgl[])  [unwired: 1 in]
        n91 = Bundle("Data P1"=w210, "Data P1"=w212) -> ()  [unwired: 1 in, 1 out]
        n92 = Build Array (concatenate)(w216, w210) -> (w220:sgl[])
        n93 = Build Array (concatenate)(w215, w213) -> (w219:sgl[])
        n94 = Bundle(w220, w219) -> (w217:cluster{sgl[], sgl[]})  [unwired: 1 in]
        n95 = Build Array(w217) -> (w211:cluster{sgl[], sgl[]}[])
      }
      frame "Idc" {
        n96 = Index Array(array=w231, index (col)=0 ("Index")) -> (element=w235:sgl[])  [unwired: 1 in]
        n97 = Index Array(array=w231, index (col)=2 ("Index")) -> (element=w234:sgl[])  [unwired: 1 in]
        n98 = Bundle("Data P1"=w228, "Data P1"=w229) -> ()  [unwired: 1 in, 1 out]
        n99 = Build Array (concatenate)(w235, w228) -> (w233:sgl[])
        n100 = Build Array (concatenate)(w234, w227) -> (w232:sgl[])
        n101 = Bundle(w233, w232) -> (w238:cluster{sgl[], sgl[]})  [unwired: 1 in]
        n102 = Build Array(w238) -> (w230:cluster{sgl[], sgl[]}[])
      }
      frame "E range" {
        n103 = Bundle("Data P1"=w247, "Data P1"=w244) -> (w246:cluster{"Data P1":sgl[], "Data P1":sgl[]})  [unwired: 1 in]
        n104 = Bundle("Data P1"=w247, "Data P1"=w245) -> ()  [unwired: 1 in, 1 out]
        n105 = Build Array(w246) -> (w243:cluster{"Data P1":sgl[], "Data P1":sgl[]}[])
      }
      frame "I range" {
        n106 = Bundle("Data P1"=w255, "Data P1"=w256) -> (w254:cluster{"Data P1":sgl[], "Data P1":sgl[]})  [unwired: 1 in]
        n107 = Build Array(w254) -> (w253:cluster{"Data P1":sgl[], "Data P1":sgl[]}[])
      }
      frame "f(t)" {
        n108 = Bundle("Data P1"=w265, "Data P1"=w264) -> (w263:cluster{"Data P1":sgl[], "Data P1":sgl[]})  [unwired: 1 in]
        n109 = Build Array(w263) -> (w262:cluster{"Data P1":sgl[], "Data P1":sgl[]}[])
      }
      frame "theta" {
        n110 = Divide(x=w272, y=6.283185307179586) -> (x/y=w277:dbl[])
        n111 = Divide(x=w273, y=6.283185307179586) -> (x/y=w285:dbl[])
        n112 = Multiply(x=w277, y=360) -> (x*y=w279:dbl[])
        n113 = Multiply(x=w285, y=360) -> (x*y=w282:dbl[])
        n114 = Bundle("Data P1"=w275, w282) -> (w274:cluster{"Data P1":sgl[], dbl[]})  [unwired: 1 in]
        n115 = Bundle("Data P1"=w275, w279) -> ()  [unwired: 1 in, 1 out]
        n116 = Build Array(w274) -> (w271:cluster{"Data P1":sgl[], dbl[]}[])
      }
    }
    "XY Graph" <- w111
    n117 = property on="XY Graph" class="XYGraph (strict)"("X Scale.Name Label.Text"=w144) -> ()  [unwired: 2 in, 2 out]
    n118 = property on="XY Graph" class="XYGraph (strict)"("Y Scale.Name Label.Text"=w147) -> ()  [unwired: 2 in, 2 out]
    n119 = property on="XY Graph" class="XYGraph (strict)"("Y Scale.Mapping Mode"=w132) -> ()  [unwired: 2 in, 2 out]
    n120 = property on="XY Graph" class="XYGraph (strict)"("X Scale.Mapping Mode"=w141) -> ()  [unwired: 2 in, 2 out]
    n121 = property on="XY Graph" class="XYGraph (strict)"("Y Scale.Flipped"=w142) -> ()  [unwired: 2 in, 2 out]
    n122 = local read "Exit 2"() -> (w140:bool)
  }
  n123 = call "disconnect.vi"("error in (no error)"=w13, "ID"=w2) -> ()  [unwired: 9 in, 1 out]
